vi "XYZ Stop.vi"(8 "error in (no error)":errorcluster, 11 "LSID":i32) -> (0 "error out":errorcluster)   [LabVIEW 2014]
uses:
  <userlib>/Tango_DLL/Tango_DLL.lvlib
panel:
  # "LICENSED MATERIALS – PROPERTY OF IBM\nCopyright IBM Corp. 2016,\nALL RIGHTS RESERVED"
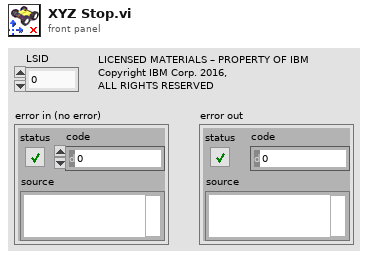
[diagram p1: front panel]
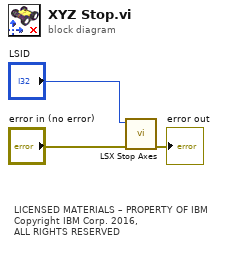
[diagram p0: block diagram]
diagram:
  # "LICENSED MATERIALS – PROPERTY OF IBM\nCopyright IBM Corp. 2016,\nALL RIGHTS RESERVED"
  n1 = call <userlib>:"LSX Stop Axes.vi"("error in (no error)"="error in (no error)", "lLSID"="LSID") -> ("error out"=→"error out":errorcluster)  [unwired: 8 in, 1 out]
